vi "Generate Bezier Spline.vi"(9 "percision":dbl=0.01, 10 "starting orientation":dbl, 11 "waypoints":cluster{dbl, dbl}[](array[cluster])) -> (0 "cubic spline ctrl pts":cluster{dbl, dbl}[][](array[cluster]), 1 "Tangents":cluster{dbl, dbl}[](array[cluster]), 2 "ctrl pts":cluster{dbl, dbl}[][](array[cluster]), 3 "bezier spline":T1)   [LabVIEW 2019]
uses:
  Types/Bezier Spline.ctl
panel:
  out "Numeric 2":dbl
  out "Numeric":dbl
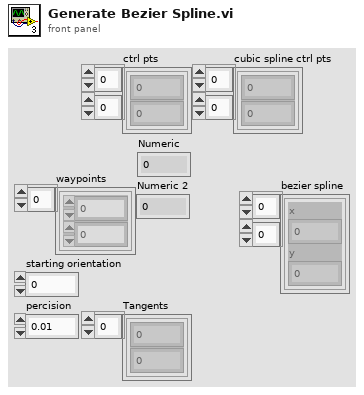
[diagram p1: front panel]
types:
  T1 = typedef "Bezier Spline.ctl" = cluster{"x":dbl, "y":dbl}[][]
  T2 = typedef "Bezier Curve.ctl" = cluster{"x":dbl, "y":dbl}[]
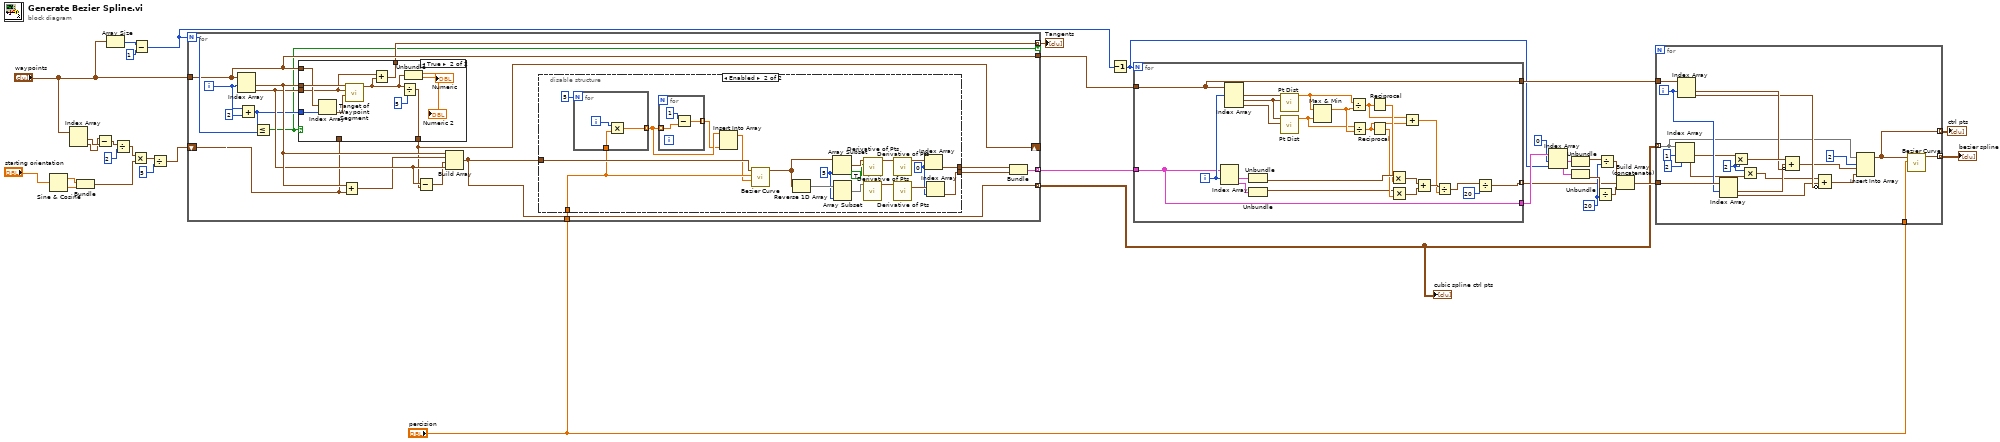
[diagram p0: block diagram]
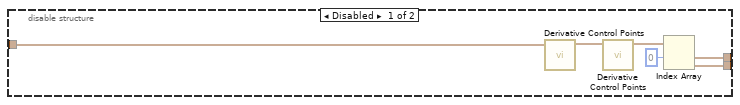
[diagram p2: hidden frame]
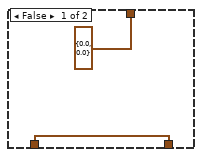
[diagram p3: hidden frame]
diagram:
  w6 = 20
  n1 = Sine & Cosine(0:"starting orientation") -> (1:w32:dbl, 2:w33:dbl)
  n2 = Index Array(array="waypoints") -> (element #1=w30:cluster{dbl, dbl}, element #2=w29:cluster{dbl, dbl})  [unwired: 2 in]
  n3 = Bundle(w32, w33) -> (w25:cluster{dbl, dbl})  [unwired: 1 in]
  n4 = Subtract(x=w29, y=w30) -> (x-y=w28:cluster{dbl, dbl})
  n5 = Array Size(array="waypoints") -> (size(s)=w36:i32)
  n6 = Divide(x=w28, y=u16 2) -> (x/y=w26:cluster{dbl, dbl})
  n7 = Multiply(x=w26, y=w25) -> (x*y=w24:cluster{dbl, dbl})
  n8 = Subtract(x=w36, y=1) -> (x-y=w19:i32)
  n9 = Divide(x=w24, y=u16 5) -> (x/y=w22:cluster{dbl, dbl})
  n10 = for {
    N: w19 -> [w43]
    tunnel: "waypoints" -> [w42]
    shift-right: [w41] -> _
    shift-left: w22 -> [w45]
    tunnel: [w40] -> w15 mode=indexing
    tunnel: [w48] -> w21 mode=indexing
    tunnel: [w42] -> w20
    tunnel: "percision" -> [w39]
    tunnel: [w38] -> w1 mode=indexing if=w37
    i -> [w47]
    n11 = Index Array(array=w42, index #1=w47) -> (element #1=w54:cluster{dbl, dbl}, element #2=w53:cluster{dbl, dbl})  [unwired: 1 in]
    n12 = Add(x=w47, y=2) -> (x+y=w44:i32)
    n13 = Less Or Equal?(x=w44, y=w43) -> (x <= y?=w37:bool)
    n14 = case shown="True" w37 {
      tunnel: w54 -> [_ w98]
      tunnel: w53 -> [_ w89]
      tunnel: [w87 w96] -> w41
      tunnel: w44 -> [_ w95]
      tunnel: w42 -> [_ w94]
      tunnel: w45 -> [w87 _]
      tunnel: [cluster{dbl, dbl} {0.0, 0.0} ("T_i") w88] -> w38
      frame False {
      }
      frame True {
        n15 = Index Array(array=w94, index=w95) -> (element=w93:cluster{dbl, dbl})
        n16 = call "Tanget of Waypoint Segment.vi"("point c"=w93, "point b"=w89, "point a"=w98) -> ("T_i"=w90:cluster{dbl, dbl})  [unwired: 8 in]
        n17 = Add(x=w89, y=w90) -> (x+y=w88:cluster{dbl, dbl})
        n18 = Divide(x=w90, y=u16 5) -> (x/y=w96:cluster{dbl, dbl})
        n19 = Unbundle(w90) -> (→"Numeric":dbl, →"Numeric 2":dbl)
      }
    }
    n20 = Add(x=w54, y=w45) -> (x+y=w52:cluster{dbl, dbl})
    n21 = Subtract(x=w53, y=w41) -> (x-y=w51:cluster{dbl, dbl})
    n22 = Build Array(w54, w52, w51, w53) -> (w40:cluster{dbl, dbl}[])
    n23 = disable-structure shown="Enabled" {
      disable-tunnel: w40 -> [w59 w67]
      disable-tunnel: [w56 w70] -> w50
      disable-tunnel: [w55 w69] -> w49
      disable-tunnel: w39 -> [_ w65]
      frame Disabled {
        n24 = call "Derivative Control Points.vi"("ctrl points"=w59) -> ("d ctrl pts"=w60:cluster{dbl, dbl}[])  [unwired: 10 in]
        n25 = call "Derivative Control Points.vi"("ctrl points"=w60) -> ("d ctrl pts"=w58:cluster{dbl, dbl}[])  [unwired: 10 in]
        n26 = Index Array(array=w58, index #1=0 ("index")) -> (element #1=w56:cluster{dbl, dbl}, element #2=w55:cluster{dbl, dbl})  [unwired: 1 in]
      }
      frame Enabled {
        w72 = 0 ("index")
        w71 = 5 ("length")
        n27 = for {
          N: 5 -> [_]
          tunnel: w65 -> [w84]
          tunnel: [w83] -> w62 mode=indexing
          i -> [w85]
          n28 = Multiply(x=w85, y=w84) -> (x*y=w83:dbl)
        }
        n29 = for {
          tunnel: w62 -> [w82] mode=indexing
          tunnel: [w80] -> w61 mode=indexing
          n30 = Subtract(x=1 ("length"), y=w82) -> (x-y=w80:dbl)
        }
        n31 = Insert Into Array(array=w62, new element=w61) -> (w64:dbl[])  [unwired: 1 in]
        n32 = call "Bezier Curve.vi"("position"=w64, "percision"=w65, "ctrl points"=w67) -> ("curve"=w63:T2)  [unwired: 8 in]
        n33 = Reverse 1D Array(array=w63) -> (reversed array=w79:T2)
        n34 = Array Subset(array=w63, length=w71) -> (w78:T2)  [unwired: 1 in]
        n35 = Array Subset(array=w79, length=w71) -> (w76:T2)  [unwired: 1 in]
        n36 = call "Derivative of Pts.vi"("pts"=w76) -> ("pts out"=w75:cluster{dbl, dbl}[])  [unwired: 10 in]
        n37 = call "Derivative of Pts.vi"("fix first pt?"=TRUE, "pts"=w78) -> ("pts out"=w77:cluster{dbl, dbl}[])  [unwired: 9 in]
        n38 = call "Derivative of Pts.vi"("pts"=w77) -> ("pts out"=w74:cluster{dbl, dbl}[])  [unwired: 10 in]
        n39 = call "Derivative of Pts.vi"("pts"=w75) -> ("pts out"=w73:cluster{dbl, dbl}[])  [unwired: 10 in]
        n40 = Index Array(array=w74, index=w72) -> (element=w70:cluster{dbl, dbl})
        n41 = Index Array(array=w73, index=w72) -> (element=w69:cluster{dbl, dbl})
      }
    }
    n42 = Bundle(w50, w49) -> (w48:cluster{cluster{dbl, dbl}, cluster{dbl, dbl}})  [unwired: 1 in]
  }
  "cubic spline ctrl pts" <- w15
  "Tangents" <- w1
  n43 = Decrement(x=w19) -> (x-1=w11:i32)
  n44 = for {
    N: w11 -> [_]
    tunnel: w21 -> [w113]
    tunnel: w20 -> [w112]
    tunnel: [w102] -> w2 mode=indexing
    tunnel: [w113] -> w18
    tunnel: [w112] -> w14
    i -> [w122]
    n45 = Index Array(array=w113, index #1=w122) -> (element #1=w121:cluster{cluster{dbl, dbl}, cluster{dbl, dbl}}, element #2=w120:cluster{cluster{dbl, dbl}, cluster{dbl, dbl}})  [unwired: 1 in]
    n46 = Index Array(array=w112, index #1=w122) -> (element #1=w119:cluster{dbl, dbl}, element #2=w118:cluster{dbl, dbl}, element #3=w117:cluster{dbl, dbl})  [unwired: 2 in]
    n47 = Unbundle(w121) -> (w110:cluster{dbl, dbl})  [unwired: 1 out]
    n48 = Unbundle(w120) -> (w107:cluster{dbl, dbl})  [unwired: 1 out]
    n49 = call "Pt Dist.vi"("point b"=w118, "point a"=w119) -> ("dist"=w116:dbl)  [unwired: 9 in]
    n50 = call "Pt Dist.vi"("point b"=w117, "point a"=w118) -> ("dist"=w114:dbl)  [unwired: 9 in]
    n51 = Max & Min(x=w116, y=w114) -> (max(x,y)=w115:dbl)  [unwired: 1 out]
    n52 = Divide(x=w116, y=w115) -> (x/y=w101:dbl)
    n53 = Divide(x=w114, y=w115) -> (x/y=w100:dbl)
    n54 = Reciprocal(x=w101) -> (1/x=w109:dbl)
    n55 = Reciprocal(x=w100) -> (1/x=w108:dbl)
    n56 = Multiply(x=w110, y=w109) -> (x*y=w106:cluster{dbl, dbl})
    n57 = Multiply(x=w107, y=w108) -> (x*y=w105:cluster{dbl, dbl})
    n58 = Add(x=w101, y=w100) -> (x+y=w99:dbl)
    n59 = Add(x=w106, y=w105) -> (x+y=w104:cluster{dbl, dbl})
    n60 = Divide(x=w104, y=w99) -> (x/y=w103:cluster{dbl, dbl})
    n61 = Divide(x=w103, y=20) -> (x/y=w102:cluster{dbl, dbl})
  }
  n62 = Index Array(array=w18, index #1=0 ("index"), index #2=w11) -> (element #1=w17:cluster{cluster{dbl, dbl}, cluster{dbl, dbl}}, element #2=w13:cluster{cluster{dbl, dbl}, cluster{dbl, dbl}})
  n63 = Unbundle(w17) -> (w7:cluster{dbl, dbl})  [unwired: 1 out]
  n64 = Unbundle(w13) -> (w9:cluster{dbl, dbl})  [unwired: 1 out]
  n65 = Divide(x=w9, y=w6) -> (x/y=w8:cluster{dbl, dbl})
  n66 = Divide(x=w7, y=w6) -> (x/y=w5:cluster{dbl, dbl})
  n67 = Build Array (concatenate)(w5, w2, w8) -> (w16:cluster{dbl, dbl}[])
  n68 = for {
    tunnel: w16 -> [w140]
    tunnel: w15 -> [w129] mode=indexing
    tunnel: w14 -> [w141]
    tunnel: "percision" -> [w125]
    tunnel: [w124] -> w10 mode=indexing
    tunnel: [w123] -> w4 mode=indexing
    i -> [w139]
    w136 = u16 2
    n69 = Index Array(array=w129, index #1=1 ("index"), index #2=2 ("index")) -> (element #1=w138:cluster{dbl, dbl}, element #2=w137:cluster{dbl, dbl})
    n70 = Index Array(array=w141, index #1=w139) -> (element #1=w133:cluster{dbl, dbl}, element #2=w132:cluster{dbl, dbl})  [unwired: 1 in]
    n71 = Index Array(array=w140, index #1=w139) -> (element #1=w134:cluster{dbl, dbl}, element #2=w130:cluster{dbl, dbl})  [unwired: 1 in]
    n72 = Multiply(x=w138, y=w136) -> (x*y=w135:cluster{dbl, dbl})
    n73 = Multiply(x=w136, y=w137) -> (x*y=w131:cluster{dbl, dbl})
    n74 = Compound Arithmetic op=ADD(w135, w134, invert w133) -> (w128:cluster{dbl, dbl})
    n75 = Compound Arithmetic op=ADD(w131, w130, invert w132) -> (w127:cluster{dbl, dbl})
    n76 = Insert Into Array(array=w129, index=2, new element #1=w128, new element #2=w127) -> (w123:cluster{dbl, dbl}[])
    n77 = call "Bezier Curve.vi"("percision"=w125, "ctrl points"=w123) -> ("curve"=w124:T2)  [unwired: 9 in]
  }
  "bezier spline" <- w10
  "ctrl pts" <- w4
